vi "Get PK Display Name.vi"(8 "error in (no error)":errorcluster, 11 "FK Ring in":refnum<class "FK Ring.lvclass">) -> (0 "error out":errorcluster, 3 "FK Ring out":refnum<class "FK Ring.lvclass">)   [LabVIEW 2020, in "FK Ring.lvclass"]
uses:
  FK Ring.lvclass
  C:/Users/User/Desktop/Raman Program/Database OOP/source/Field/Field.lvclass
  Field.lvclass/Field.ctl
  FK Ring.lvclass/FK Ring.ctl
  Database.lvclass
  Field.lvclass
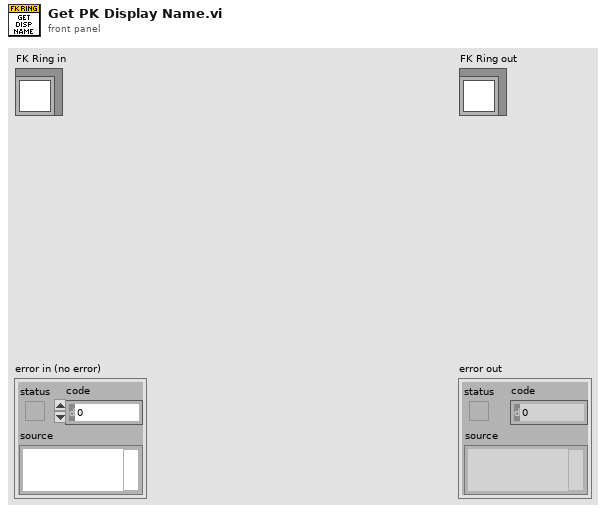
[diagram p1: front panel]
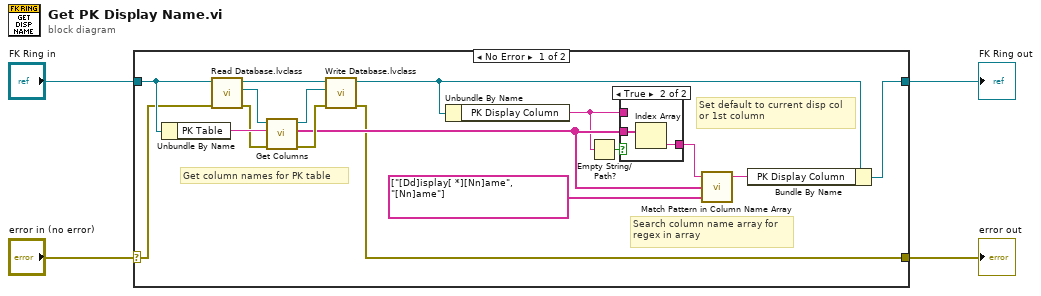
[diagram p0: block diagram]
diagram:
  n1 = case shown="No Error" "error in (no error)" {
    selector: "error in (no error)" -> [w14 w26]
    tunnel: [w5 w26] -> w3
    tunnel: [w10 w25] -> w1
    tunnel: "FK Ring in" -> [w18 w25]
    frame No Error {
      # "Search column name array for\nregex in array"
      # "Set default to current disp col\nor 1st column"
      # "Get column names for PK table"
      n2 = Unbundle By Name(w18) -> ("PK Table"=w17:string)
      n3 = call "Read Database.lvclass.vi"("error in (no error)"=w14, "Field in"=w18) -> ("error out"=w16:errorcluster, "Database.lvclass"=w20:refnum<class "Database.lvclass">, "Field out"=w21:refnum<class "FK Ring.lvclass">)  [unwired: 7 in]
      n4 = call-dynamic "Get Columns.vi"("error in (no error)"=w16, "Table Name"=w17, "Database in"=w20) -> ("error out"=w15:errorcluster, "Column Name Array"=w12:string[], "Database out"=w19:refnum<class "Database.lvclass">)  [unwired: 6 in]
      n5 = call "Write Database.lvclass.vi"("error in (no error)"=w15, "Database.lvclass"=w19, "Field in"=w21) -> ("error out"=w5:errorcluster, "Field out"=w9:refnum<class "FK Ring.lvclass">)  [unwired: 7 in]
      n6 = Unbundle By Name(w9) -> ("PK Display Column"=w7:string)
      n7 = Empty String/Path?(string/path=w7) -> (empty?=w8:bool)
      n8 = case shown="True" w8 {
        tunnel: [w22 w24] -> w13
        tunnel: w12 -> [_ w23]
        tunnel: w7 -> [w22 _]
        frame False {
        }
        frame True {
          n9 = Index Array(array=w23) -> (element=w24:string)  [unwired: 1 in]
        }
      }
      n10 = call "Match Pattern in Column Name Array.vi"("Match Pattern Regex"=string[] ["[Dd]isplay[ *][Nn]ame", "[Nn]ame"], "Column Name Array"=w12, "Not Found Name"=w13) -> ("Matching Name"=w6:string)  [unwired: 2 out]
      n11 = Bundle By Name(cluster=w9, "PK Display Column"=w6) -> (w10:refnum<class "FK Ring.lvclass">)
    }
    frame Error {
    }
  }
  "error out" <- w3
  "FK Ring out" <- w1
